vi "FTW-Subscriber-Worker.vi"(0 "Endpoint":refnum<class "FTW-Endpoint.lvclass">, 5 "Message Handler":refnum<user-event>, 7 "Queue":refnum<queue>) -> ()   [LabVIEW 2013, in "FTW-Subscriber.lvclass"]
uses:
  FTW-Subscriber.lvclass
  Message/Base/FTW-Message.lvclass
  Endpoint/FTW-Endpoint.lvclass
  Message/Lossy/FTW-Message-Lossy.lvclass
panel:
  out "Messages Received":u32
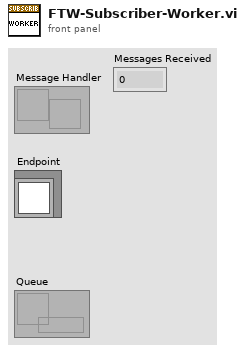
[diagram p1: front panel]
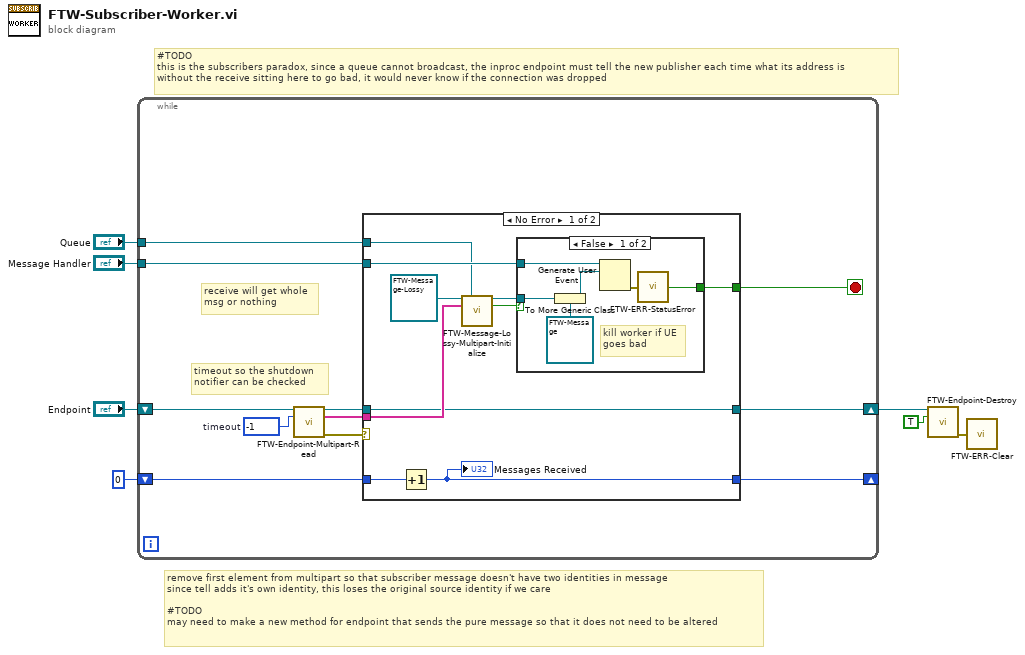
[diagram p0: block diagram]
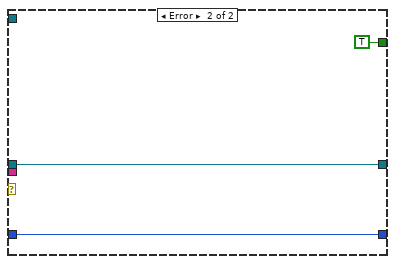
[diagram p3: hidden frame]
diagram:
  # "#TODO\nthis is the subscribers paradox, since a queue cannot broadcast, the inproc endpoint must tell the new publisher each time what its address is\nwithout the receive sitting here to go bad, it would never know if the connection was dropped"
  # "remove first element from multipart so that subscriber message doesn't have two identities in message\nsince tell adds it's own identity, this loses the original source identity if we care\n\n#TODO\nmay need to make a new method for endpoint that sends the pure message so that it does not need to be altered"
  n1 = while {
    tunnel: "Message Handler" -> [w18]
    shift-right: [w15] -> _
    shift-left: u32 0 -> [w16]
    shift-right: [w13] -> w2
    shift-left: "Endpoint" -> [w17]
    tunnel: "Queue" -> [w12]
    stop <- w14 stop-if-true
    w11 = -1  # timeout
    # "receive will get whole\nmsg or nothing"
    # "timeout so the shutdown\nnotifier can be checked"
    n2 = call-dynamic "FTW-Endpoint-Multipart-Read.vi"("FTW Endpoint"=w17, "Timeout"=w11) -> ("FTW Endpoint out"=w8:refnum<class "FTW-Endpoint.lvclass">, "Message Received"=w9:string[], "error out"=w10:errorcluster)  [unwired: 10 in, 1 out]
    n3 = case shown="No Error" w10 {
      tunnel: w18 -> [w28 _]
      tunnel: w9 -> [w23 _]
      tunnel: w16 -> [w27 w37]
      tunnel: [w26 w37] -> w15
      tunnel: w8 -> [w21 w35]
      tunnel: [w22 TRUE ("Error?")] -> w14
      tunnel: [w21 w35] -> w13
      tunnel: w12 -> [w20 _]
      frame No Error {
        n4 = Increment(x=w27) -> (x+1=w26:u32)
        "Messages Received" <- w26
        n5 = call-dynamic "FTW-Message-Lossy-Multipart-Initialize.vi"("FTW-Message-Lossy In"=refnum<class "FTW-Message-Lossy.lvclass"> refnum ("FTW Message"), "Queue"=w20, "Message Parts"=w23) -> ("FTW-Message-Lossy Out"=w25:refnum<class "FTW-Message-Lossy.lvclass">, "overflow?"=w19:bool)  [unwired: 10 in, 1 out]
        n6 = case shown="False" w19 {
          tunnel: w28 -> [w34 _]
          tunnel: w25 -> [w33 _]
          tunnel: [w31 _] -> w22
          frame False {
            # "kill worker if UE\ngoes bad"
            n7 = To More Generic Class(target class=refnum<class "FTW-Message.lvclass"> refnum ("FTW Message"), reference=w33) -> (generic class reference=w30:refnum<class "FTW-Message.lvclass">)
            n8 = Generate User Event(user event=w34, event data cluster=w30) -> (error out=w32:errorcluster)  [unwired: 2 in, 1 out]
            n9 = call "FTW-ERR-StatusError.vi"("error to check"=w32) -> ("Error?"=w31:bool)
          }
          frame True {
          }
        }
      }
      frame Error {
      }
    }
  }
  n10 = call-dynamic "FTW-Endpoint-Destroy.vi"("FTW Endpoint"=w2, "Force Destroy"=TRUE) -> ("error out"=w4:errorcluster)  [unwired: 13 in]
  n11 = call "FTW-ERR-Clear.vi"("error to snuff"=w4) -> ()  [unwired: 1 out]
